vi "Remove Header.vi"(8 "error in":errorcluster, 10 "header":string, 11 "REST Client in":refnum<class "REST Client.lvclass">) -> (0 "error out":errorcluster, 3 "REST Client out":refnum<class "REST Client.lvclass">)   [LabVIEW 2020, in "REST Client.lvlib" / "REST Client.lvclass"]
uses:
  REST Client.lvclass
  REST Client.lvclass/REST Client.ctl
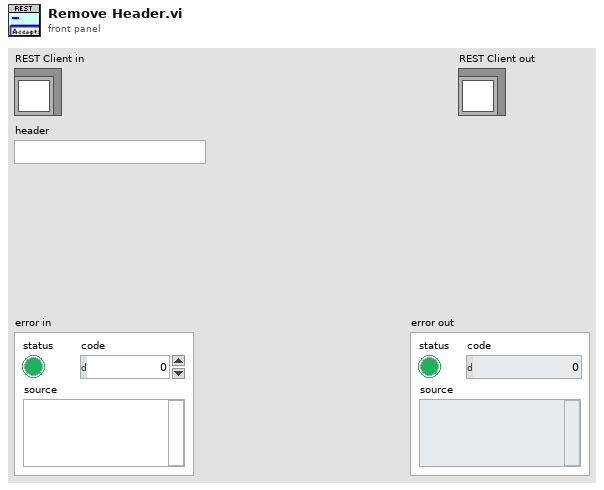
[diagram p1: front panel]
types:
  T1 = typedef "REST Client.lvlib/REST Client.lvclass/HTTP Header.ctl" = cluster{"header":string, "value":string}
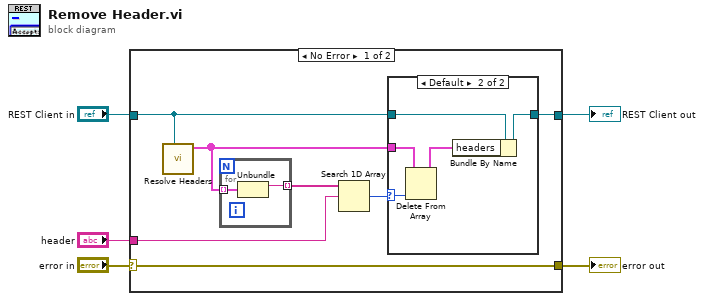
[diagram p0: block diagram]
diagram:
  n1 = case shown="No Error" "error in" {
    selector: "error in" -> [w7 w21]
    tunnel: "header" -> [w12 _]
    tunnel: "REST Client in" -> [w8 w22]
    tunnel: [w6 w22] -> w3
    tunnel: [w7 w21] -> w2
    frame No Error {
      n2 = call "Resolve Headers.vi"("REST Client in"=w8) -> ("headers out"=w9:T1[])  [unwired: 10 in]
      n3 = for {
        tunnel: w9 -> [w20] mode=indexing
        tunnel: [w19] -> w10 mode=indexing
        n4 = Unbundle(w20) -> ("header"=w19:string)  [unwired: 1 out]
      }
      n5 = Search 1D Array(1D array=w10, element=w12) -> (index of element=w11:i32)  [unwired: 1 in]
      n6 = case shown="Default" w11 {
        selector: w11 -> [_ w17]
        tunnel: w9 -> [_ w18]
        tunnel: w8 -> [w13 w14]
        tunnel: [w13 w15] -> w6
        frame -1 {
        }
        frame Default {
          n7 = Delete From Array(array=w18, index=w17) -> (array with subset deleted=w16:T1[])  [unwired: 1 in, 1 out]
          n8 = Bundle By Name(cluster=w14, "headers"=w16) -> (w15:refnum<class "REST Client.lvclass">)
        }
      }
    }
    frame Error {
    }
  }
  "error out" <- w2
  "REST Client out" <- w3
